vi "New Image (Greyscale).vi"(7 "Value (Default: 0)":u8, 8 "error in (no error)":errorcluster, 11 "Preallocated Image Size (Default 0,0)":T2) -> (0 "error out":errorcluster, 3 "New Greyscale Image":T1)   [LabVIEW 2020, in "g_ar_toolkit.image.lvlib"]
uses:
  g_ar_toolkit.image.lvlib
  g_ar_toolkit.common/Image Size (Integer).ctl
  Greyscale Image.ctl
  6598b9e0-8a08-46f5-91fd-ca1b87217137.vi
  g_ar_toolkit.common/Module Path.vi
  <vilib>/Utility/error.llb/Error Cluster From Error Code.vi
  g_ar_toolkit.common/g_ar_toolkit.common.lvlib
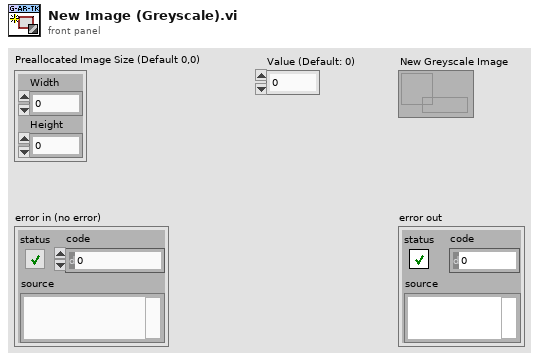
[diagram p1: front panel]
types:
  T1 = typedef "g_ar_toolkit.image.lvlib/Greyscale Image.ctl" = refnum<data-value>
  T2 = typedef "g_ar_toolkit.common.lvlib/Image Size (Integer).ctl" = cluster{"Width":u16, "Height":u16}
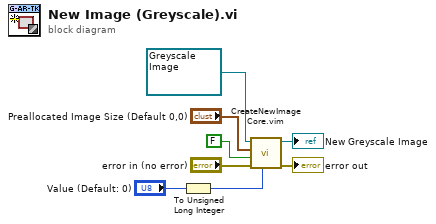
[diagram p0: block diagram]
diagram:
  n1 = To Unsigned Long Integer(number="Value (Default: 0)") -> (unsigned 32bit integer=w1:u32)
  n2 = call "CreateNewImageCore.vim"("Initial Value"=w1, "error in (no error)"="error in (no error)", "Is ARGB"=FALSE, "Preallocated Image Size"="Preallocated Image Size (Default 0,0)", "Ref Type"=T1 refnum ("EDVR")) -> ("error out"=→"error out":errorcluster, "New Reference"=→"New Greyscale Image":T1)  [unwired: 5 in]
